vi "String - Convert String Only TimeStamp.vi"(11 "YYYYmmdd_HHMMSS":string) -> (3 "YYYY-mm-dd HH:MM:SS":string)   [LabVIEW 2013]
panel:
  out "Array":string[](array[string])
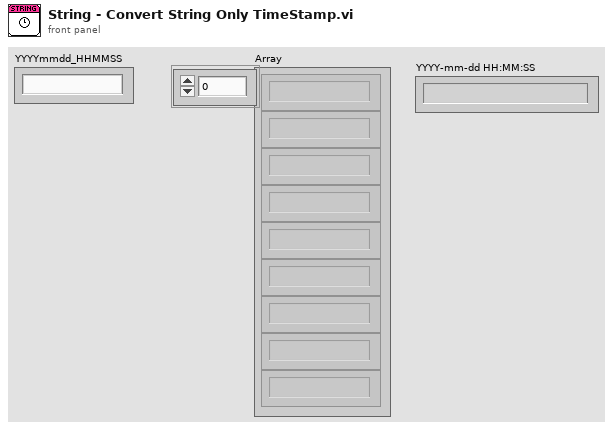
[diagram p1: front panel]
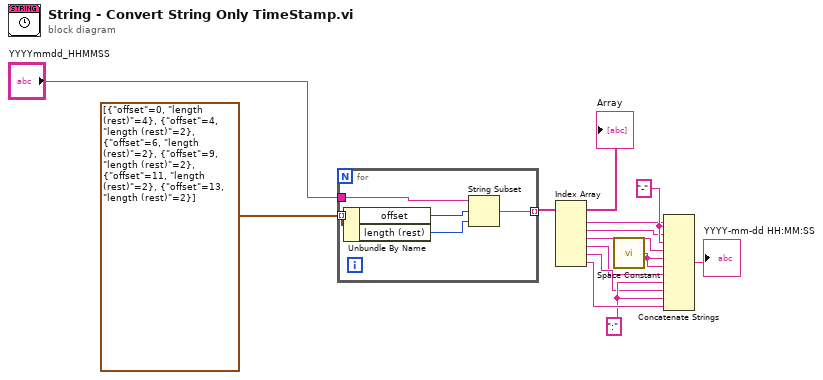
[diagram p0: block diagram]
diagram:
  w11 = ":"
  w7 = "-"
  n1 = for {
    tunnel: "YYYYmmdd_HHMMSS" -> [w18]
    tunnel: cluster{"offset":i32, "length (rest)":i32}[] [{"offset"=0, "length (rest)"=4}, {"offset"=4, "length (rest)"=2}, {"offset"=6, "length (rest)"=2}, {"offset"=9, "length (rest)"=2}, {"offset"=11, "length (rest)"=2}, {"offset"=13, "length (rest)"=2}] -> [w17] mode=indexing
    tunnel: [w14] -> w4 mode=indexing
    n2 = Unbundle By Name(w17) -> ("offset"=w16:i32, "length (rest)"=w15:i32)
    n3 = String Subset(string=w18, offset (0)=w16, length (rest)=w15) -> (substring=w14:string)
  }
  "Array" <- w4
  n4 = Index Array(array=w4) -> (element #1=w5:string, element #2=w6:string, element #3=w8:string, element #4=w9:string, element #5=w10:string, element #6=w12:string)  [unwired: 6 in]
  n5 = call <vilib>:"Space Constant.vi"() -> ("String"=w1:string)
  n6 = Concatenate Strings(w5, w7, w6, w7, w8, w1, w1, w9, w11, w10, w11, w12) -> (→"YYYY-mm-dd HH:MM:SS":string)
